vi "GFITS_AsyncMsgs.vi"(4 "max imlist size":i32=200000, 5 "asyncs":refnum<vi>, 6 "postproc":refnum<vi>, 7 "imlogs":path, 8 "imlog":bool, 9 "PPQ":refnum<queue>, 10 "imlogq":refnum<queue>, 11 "notifier in":refnum<notifier>) -> ()   [LabVIEW 2016]
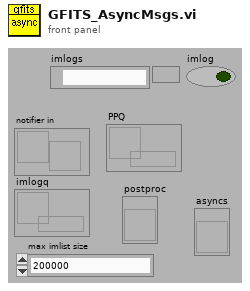
[diagram p1: front panel]
types:
  T1 = cluster{"command":string, "data":string, "responseQ":string, "nodeID":string}
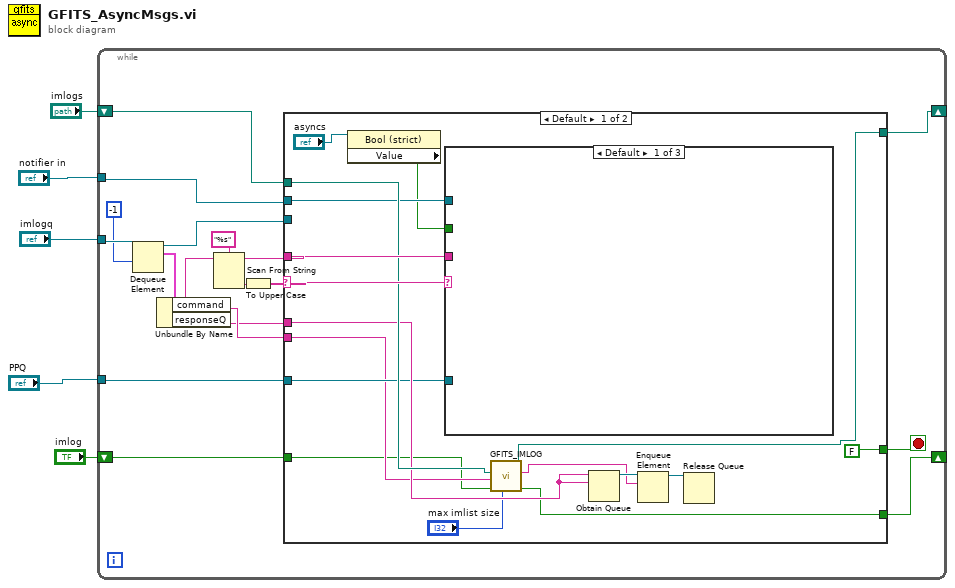
[diagram p0: block diagram]
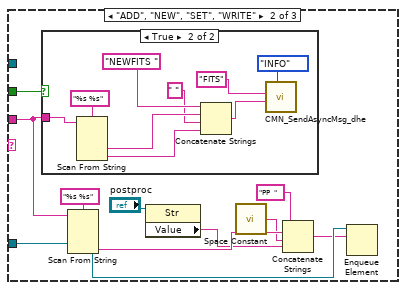
[diagram p2: hidden frame]
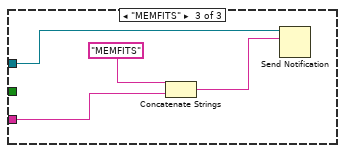
[diagram p4: hidden frame]
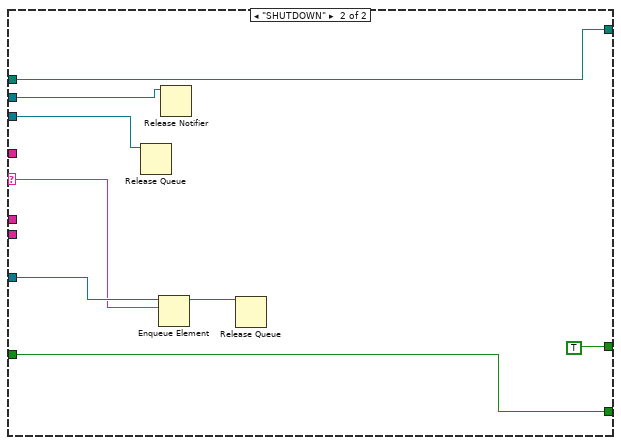
[diagram p5: hidden frame]
diagram:
  n1 = while {
    tunnel: "imlogq" -> [w22]
    tunnel: "notifier in" -> [w11]
    tunnel: "PPQ" -> [w10]
    shift-right: [w8] -> _
    shift-left: "imlogs" -> [w9]
    shift-right: [w7] -> _
    shift-left: "imlog" -> [w6]
    stop <- w18 stop-if-true
    n2 = Dequeue Element(queue=w22, timeout in ms (-1)=-1) -> (queue out=w17:refnum<queue>, element=w14:T1)  [unwired: 1 in, 2 out]
    n3 = Unbundle By Name(w14) -> ("command"=w13:string, "responseQ"=w12:string)
    n4 = Scan From String(format string="%s", input string=w13) -> (remaining string=w19:string, output 1=w20:string)  [unwired: 2 in, 3 out]
    n5 = To Upper Case(1:w20) -> (0:w15:string)
    n6 = case shown="Default" w15 {
      selector: w15 -> [w39 w65]
      tunnel: w19 -> [w37 _]
      tunnel: w9 -> [w36 w64]
      tunnel: w13 -> [w28 _]
      tunnel: [FALSE TRUE] -> w18
      tunnel: w17 -> [_ w69]
      tunnel: w12 -> [w35 _]
      tunnel: w11 -> [w31 w68]
      tunnel: w10 -> [w29 w67]
      tunnel: [w25 w64] -> w8
      tunnel: [w24 w63] -> w7
      tunnel: w6 -> [w23 w63]
      frame Default {
        n7 = property on="Property Node" class="Bool (strict)"(reference="asyncs") -> ("Value"=w30:bool)  [unwired: 1 in, 2 out]
        n8 = case shown="Default" w39 {
          tunnel: w37 -> [_ w48 w61]
          tunnel: w30 -> [_ w49 _]
          tunnel: w31 -> [_ _ w60]
          tunnel: w29 -> [_ w46 _]
          frame Default {
          }
          frame "ADD", "NEW", "SET", "WRITE" {
            n9 = case shown="True" w49 {
              tunnel: w48 -> [_ w54]
              frame False {
              }
              frame True {
                n10 = Scan From String(format string="%s %s", input string=w54) -> (output 1=w52:string, output 2=w51:string)  [unwired: 2 in, 5 out]
                n11 = Concatenate Strings("NEWFITS " ("string"), w52, " " ("string"), w51) -> (w55:string)
                n12 = call "CMN_SendAsyncMsg_dhe.vi"("type"=enum16{"ERROR", "WARNING", "INFO", "CHANGED"}."INFO", "Message"=w55, "device"="FITS") -> ()  [unwired: 1 in, 8 out]
              }
            }
            n13 = Scan From String(format string="%s %s", input string=w48) -> (output 2=w44:string)  [unwired: 2 in, 6 out]
            n14 = property on="Property Node" class="Str"(reference="postproc") -> ("Value"=w40:string)  [unwired: 1 in, 2 out]
            n15 = call <vilib>:"Space Constant.vi"() -> ("String"=w43:string)
            n16 = Concatenate Strings("PP  " ("format string"), w44, w43, w40) -> (w42:string)
            n17 = Enqueue Element(queue=w46, element=w42) -> ()  [unwired: 1 in, 4 out]
          }
          frame "MEMFITS" {
            n18 = Concatenate Strings("MEMFITS" ("string"), w61) -> (w59:string)
            n19 = Send Notification(notification=w59, notifier=w60) -> ()  [unwired: 1 in, 2 out]
          }
        }
        n20 = call "GFITS_IMLOG.vi"("max bytes size"="max imlist size", "log"=w23, "command"=w28, "imlogpath"=w36) -> ("log out"=w24:bool, "answer"=w33:string, "imlogpath out"=w25:path)  [unwired: 5 out]
        n21 = Obtain Queue(name (unnamed)=w35, element data type=w35) -> (queue out=w34:refnum<queue>)  [unwired: 3 in, 2 out]
        n22 = Enqueue Element(queue=w34, element=w33) -> (queue out=w32:refnum<queue>)  [unwired: 1 in, 3 out]
        n23 = Release Queue(queue=w32) -> ()  [unwired: 1 in, 4 out]
      }
      frame "SHUTDOWN" {
        n24 = Release Queue(queue=w69) -> ()  [unwired: 1 in, 4 out]
        n25 = Enqueue Element(queue=w67, element=w65) -> (queue out=w66:refnum<queue>)  [unwired: 1 in, 3 out]
        n26 = Release Notifier(notifier=w68) -> ()  [unwired: 1 in, 4 out]
        n27 = Release Queue(queue=w66) -> ()  [unwired: 1 in, 4 out]
      }
    }
  }
